vi "MGCC_FntStaMach_Error_State_Control_main_phasetwo_opalRT.vi"() -> ()   [LabVIEW 2016]
uses:
  Finite State Machine (He Yin)/Sub-VIs/MGCC_FntStaMach_gobal.vi
  Sub_VIs/Fault_Abnormal_state.vi
panel:
  out "appended array":errorcluster[](array[cluster])
  in  "Boolean 2":bool
  out "Boolean":bool
  out "result":bool
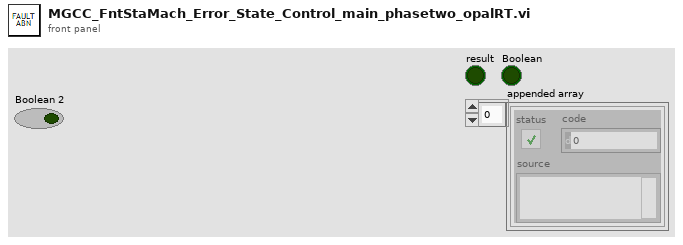
[diagram p1: front panel]
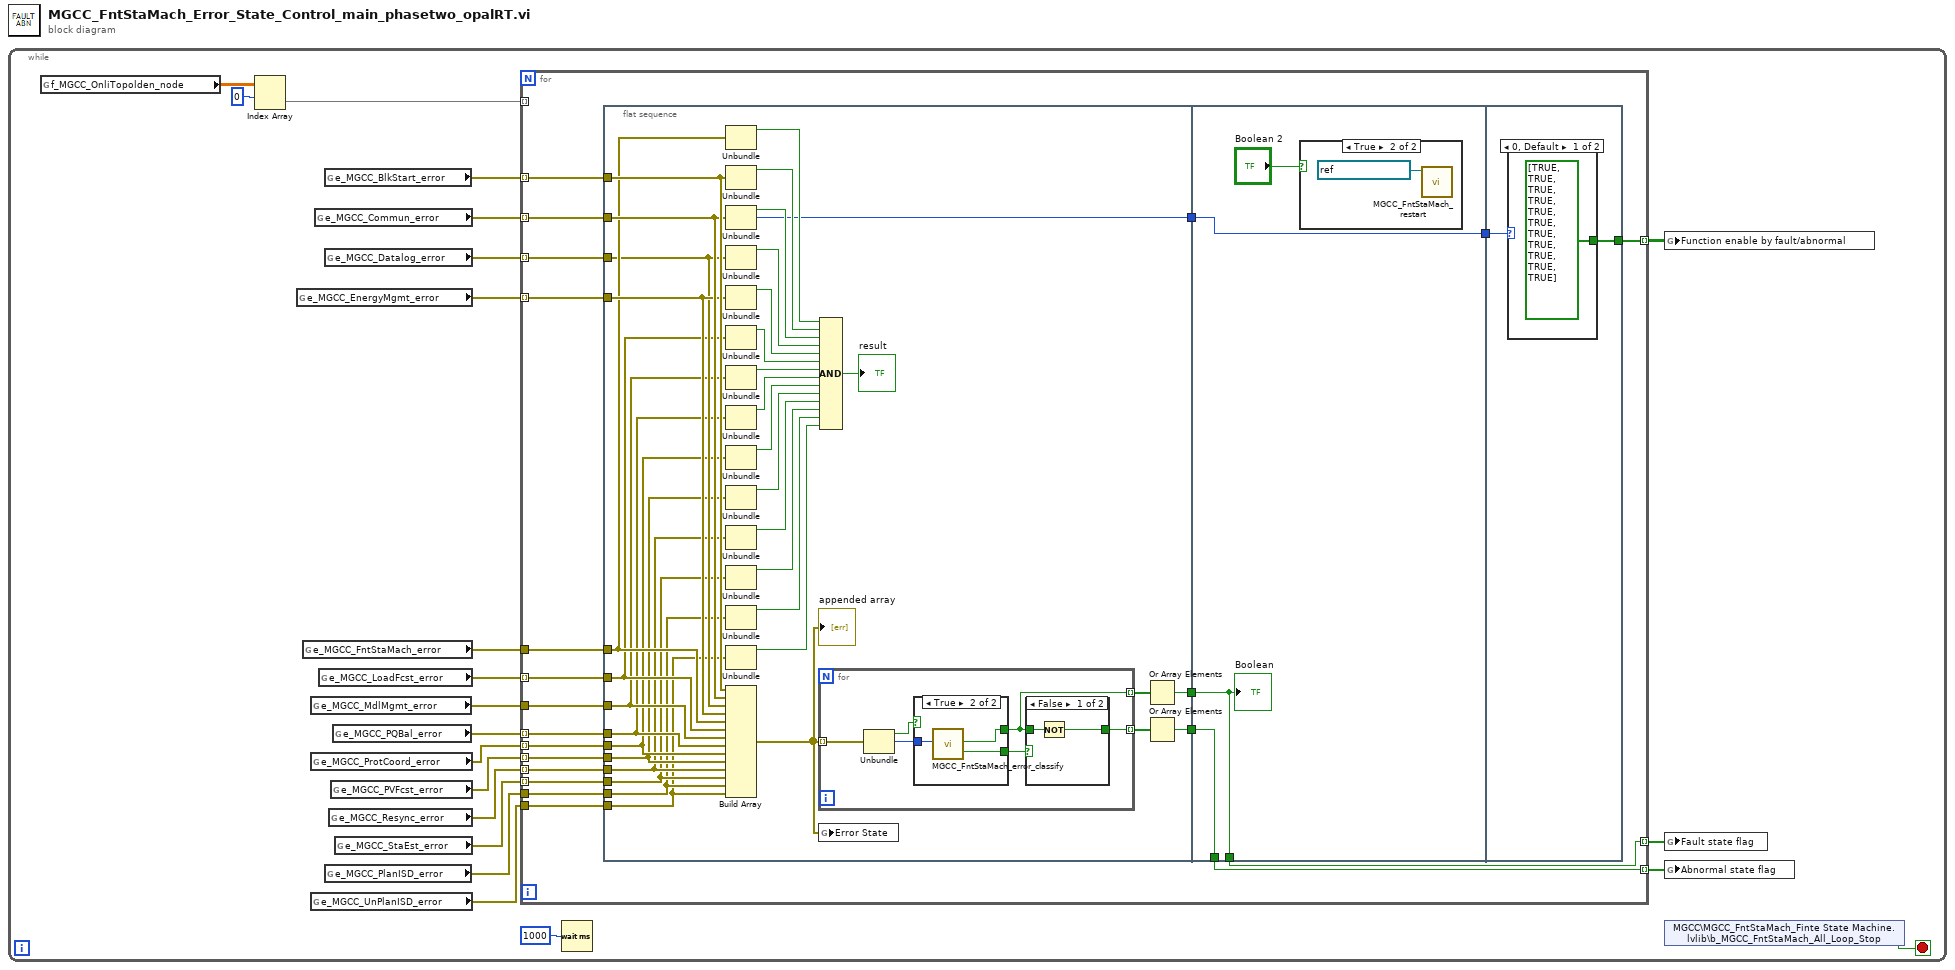
[diagram p0: block diagram]
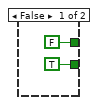
[diagram p2: hidden frame]
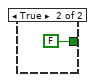
[diagram p3: hidden frame]
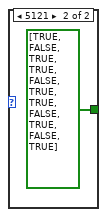
[diagram p5: hidden frame]
diagram:
  n1 = while {
    stop <- w22 stop-if-true
    n2 = global read "MGCC_FntStaMach_gobal.vi" "f_MGCC_OnliTopolden_node"() -> (w21:dbl[][])
    n3 = Index Array(array=w21, index (row)=0) -> (element=w19:dbl[])  [unwired: 1 in]
    n4 = global read "Fault_Abnormal_state.vi" "e_MGCC_EnergyMgmt_error"() -> (w16:errorcluster[])
    n5 = global read "Fault_Abnormal_state.vi" "e_MGCC_FntStaMach_error"() -> (w15:errorcluster)
    n6 = global read "Fault_Abnormal_state.vi" "e_MGCC_MdlMgmt_error"() -> (w12:errorcluster)
    n7 = global read "Fault_Abnormal_state.vi" "e_MGCC_ProtCoord_error"() -> (w10:errorcluster[])
    n8 = global read "Fault_Abnormal_state.vi" "e_MGCC_UnPlanISD_error"() -> (w1:errorcluster)
    n9 = global read "Fault_Abnormal_state.vi" "e_MGCC_Commun_error"() -> (w17:errorcluster[])
    n10 = global read "Fault_Abnormal_state.vi" "e_MGCC_LoadFcst_error"() -> (w13:errorcluster[])
    n11 = global read "Fault_Abnormal_state.vi" "e_MGCC_BlkStart_error"() -> (w18:errorcluster[])
    n12 = global read "Fault_Abnormal_state.vi" "e_MGCC_Datalog_error"() -> (w14:errorcluster[])
    n13 = global read "Fault_Abnormal_state.vi" "e_MGCC_PlanISD_error"() -> (w2:errorcluster)
    n14 = global read "Fault_Abnormal_state.vi" "e_MGCC_Resync_error"() -> (w8:errorcluster[])
    n15 = global read "Fault_Abnormal_state.vi" "e_MGCC_PVFcst_error"() -> (w9:errorcluster[])
    n16 = global read "Fault_Abnormal_state.vi" "e_MGCC_PQBal_error"() -> (w11:errorcluster[])
    n17 = global read "Fault_Abnormal_state.vi" "e_MGCC_StaEst_error"() -> (w7:errorcluster[])
    n18 = for {
      tunnel: w19 -> [_] mode=indexing
      tunnel: w18 -> [w39] mode=indexing
      tunnel: w17 -> [w38] mode=indexing
      tunnel: w16 -> [w37] mode=indexing
      tunnel: w15 -> [w36]
      tunnel: w14 -> [w35] mode=indexing
      tunnel: w13 -> [w34] mode=indexing
      tunnel: w12 -> [w33]
      tunnel: w11 -> [w32] mode=indexing
      tunnel: w10 -> [w31] mode=indexing
      tunnel: w9 -> [w30] mode=indexing
      tunnel: w8 -> [w29] mode=indexing
      tunnel: w7 -> [w28] mode=indexing
      tunnel: [w27] -> w6 mode=indexing
      tunnel: [w26] -> w5 mode=indexing
      tunnel: [w25] -> w4 mode=indexing
      tunnel: w2 -> [w24]
      tunnel: w1 -> [w23]
      n19 = flat-sequence {
        tunnel: [w62] -> w43
        tunnel: [w63] -> w42
        tunnel: [w60] -> w41
        tunnel: w39 -> [w59]
        tunnel: w38 -> [w58]
        tunnel: w37 -> [w57]
        tunnel: w36 -> [w56]
        tunnel: w35 -> [w55]
        tunnel: w34 -> [w54]
        tunnel: w33 -> [w53]
        tunnel: w32 -> [w52]
        tunnel: w31 -> [w51]
        tunnel: w30 -> [w50]
        tunnel: w29 -> [w49]
        tunnel: w28 -> [w48]
        tunnel: w24 -> [w47]
        tunnel: w23 -> [w44]
        tunnel: w43 -> [w94]
        tunnel: w42 -> [w93]
        tunnel: [w95] -> w40
        tunnel: w41 -> [w95]
        tunnel: [w94] -> w26
        tunnel: [w93] -> w25
        tunnel: w40 -> [w99]
        tunnel: [w98] -> w27
        frame #0 {
          n20 = Unbundle(w56) -> ("status"=w78:bool)  [unwired: 2 out]
          n21 = Unbundle(w59) -> ("status"=w77:bool)  [unwired: 2 out]
          n22 = Unbundle(w58) -> ("status"=w76:bool, "code"=w60:i32)  [unwired: 1 out]
          n23 = Unbundle(w55) -> ("status"=w75:bool)  [unwired: 2 out]
          n24 = Unbundle(w57) -> ("status"=w74:bool)  [unwired: 2 out]
          n25 = Unbundle(w54) -> ("status"=w73:bool)  [unwired: 2 out]
          n26 = Unbundle(w53) -> ("status"=w72:bool)  [unwired: 2 out]
          n27 = Unbundle(w52) -> ("status"=w71:bool)  [unwired: 2 out]
          n28 = Unbundle(w51) -> ("status"=w70:bool)  [unwired: 2 out]
          n29 = Unbundle(w50) -> ("status"=w69:bool)  [unwired: 2 out]
          n30 = Unbundle(w49) -> ("status"=w68:bool)  [unwired: 2 out]
          n31 = Unbundle(w48) -> ("status"=w67:bool)  [unwired: 2 out]
          n32 = Unbundle(w47) -> ("status"=w46:bool)  [unwired: 2 out]
          n33 = Unbundle(w44) -> ("status"=w45:bool)  [unwired: 2 out]
          n34 = Build Array(w59, w58, w55, w57, w56, w54, w53, w52, w51, w50, w49, w48, w47, w44) -> (w61:errorcluster[])
          "appended array" <- w61
          n35 = for {
            tunnel: w61 -> [w82] mode=indexing
            tunnel: [w81] -> w65 mode=indexing
            tunnel: [w80] -> w64 mode=indexing
            n36 = Unbundle(w82) -> ("status"=w79:bool, "code"=w84:i32)  [unwired: 1 out]
            n37 = case shown="True" w79 {
              tunnel: w84 -> [_ w89]
              tunnel: [TRUE ("No error") w88] -> w83
              tunnel: [FALSE ("Error state") w87] -> w81
              frame False {
              }
              frame True {
                n38 = call "MGCC_FntStaMach_error_classify.vi"("Error"=w89) -> ("Error state"=w87:bool, "No error"=w88:bool)  [unwired: 17 in]
              }
            }
            n39 = case shown="False" w83 {
              tunnel: [w90 FALSE] -> w80
              tunnel: w81 -> [w91 _]
              frame False {
                n40 = Not(x=w91) -> (.not. x?=w90:bool)
              }
              frame True {
              }
            }
          }
          n41 = global write "Fault_Abnormal_state.vi" "Error State"(w61) -> ()
          n42 = Compound Arithmetic op=AND(w78, w77, w76, w75, w74, w73, w72, w71, w70, w69, w68, w67, w46, w45) -> (→"result":bool)
          n43 = Or Array Elements(Boolean array=w65) -> (logical OR=w62:bool)
          n44 = Or Array Elements(Boolean array=w64) -> (logical OR=w63:bool)
        }
        frame #1 {
          n45 = case shown="True" "Boolean 2" {
            frame False {
            }
            frame True {
              n46 = call "MGCC_FntStaMach_restart.vi"("Session in"=refnum<k21> "48.26.87.212") -> ()  [unwired: 8 in, 3 out]
            }
          }
          "Boolean" <- w94
        }
        frame #2 {
          n47 = case shown="0, Default" w99 {
            tunnel: [bool[] [TRUE, TRUE, TRUE, TRUE, TRUE, TRUE, TRUE, TRUE, TRUE, TRUE, TRUE] ("Function enable by fault/abnormal") bool[] [TRUE, FALSE, TRUE, TRUE, FALSE, TRUE, TRUE, FALSE, TRUE, FALSE, TRUE] ("Function enable by fault/abnormal")] -> w98
            frame 0, Default {
            }
            frame 5121 {
            }
          }
        }
      }
    }
    n48 = Wait (ms)(milliseconds to wait=u32 1000) -> ()  [unwired: 1 out]
    n49 = global write "Fault_Abnormal_state.vi" "Function enable by fault/abnormal"(w6) -> ()
    n50 = global write "Fault_Abnormal_state.vi" "Fault state flag"(w5) -> ()
    n51 = global write "Fault_Abnormal_state.vi" "Abnormal state flag"(w4) -> ()
    n52 = shared-variable "MGCC\\MGCC_FntStaMach_Finte State Machine.lvlib\\b_MGCC_FntStaMach_All_Loop_Stop"() -> (w22:bool)  [unwired: 1 in, 1 out]
  }
